vi "transconductance.vi"(6 "reverse flattening array?":bool, 10 "load data from file?":bool=TRUE, 11 "New Files to Process":string="\\G:\\My Drive\\ansom\\Data\\MNK\\SA03018F.20171127\\8 - sweep B, Vsg lockin\n\\G:\\My Drive\\ansom\\Data\\MNK\\SA03018F.20171127\\8A - sweep B, Vsg lockin\n\\G:\\My Drive\\ansom\\Data\\MNK\\SA03018F.20171127\\11 - sweep B, Vsg lockin\n\\G:\\My Drive\\ansom\\Data\\MNK\\SA03018F.20171127\\14 - sweep B, Vsg lockin, control\n\\G:\\My Drive\\ansom\\Data\\MNK\\SA03018F.20171127\\16A - sweep B, Vsg lockin, control\n\\G:\\My Drive\\ansom\\Data\\MNK\\SA03018F.20171127\\17A - sweep B, Vsg lockin, superlattice\nG:\\My Drive\\ansom\\Data\\MNK\\SA03018F.20171127\\17B - sweep B, Vsg lockin, superlattice\n\\G:\\My Drive\\ansom\\Data\\MNK\\SA03018F.20171127\\20A- sweep B, Vsg lockin, superlattice\n\\G:\\My Drive\\ansom\\Data\\MNK\\SA03018F.20171127\\20B- sweep B, Vsg lockin, superlattice\n\\G:\\My Drive\\ansom\\Data\\MNK\\SA03018F.20171127\\21 - sweep B, Vsg lockin, superlattice\n\\G:\\My Drive\\ansom\\Data\\MNK\\SA03018F.20171127\\27 - sweep B, Vsg lockin, superlattice\n\\G:\\My Drive\\ansom\\Data\\MNK\\SA03018F.20171127\\28 - sweep B, Vsg lockin, superlattice\n\\G:\\My Drive\\ansom\\Data\\MNK\\SA03018F.20171127\\30 A- sweep B, Vsg lockin, superlattice #1, 10 deg") -> (0 "N Array":T3(array[cluster])=[{"N1"=-18.0066, "N2"=0.0, "N3"=0.00010031838163786089, "N4"=-8.934251517959054e-06}, {"N1"=-18.0066, "N2"=0.0, "N3"=0.00010015710688317914, "N4"=-8.760468576758047e-06}, {"N1"=-17.8982, "N2"=0.0, "N3"=0.00010015658578170592, "N4"=-8.792187056308865e-06}, {"N1"=-17.7321, "N2"=0.0, "N3"=0.00010023617314889044, "N4"=-8.779868263484922e-06}, {"N1"=-17.5726, "N2"=0.0, "N3"=0.00010019995511560665, "N4"=-8.84165774395135e-06}, {"N1"=-17.4134, "N2"=0.0, "N3"=0.00010003346980786668, "N4"=-8.782458591171434e-06}, {"N1"=-17.2466, "N2"=0.0, "N3"=0.0001001851515834062, "N4"=-8.812405740457855e-06}, {"N1"=-17.0876, "N2"=0.0, "N3"=9.996424752835683e-05, "N4"=-8.954710552212481e-06}, {"N1"=-16.9281, "N2"=0.0, "N3"=0.00010007646623264942, "N4"=-8.854481733875301e-06}, {"N1"=-16.7606, "N2"=0.0, "N3"=0.00010004679822862351, "N4"=-8.981470131499153e-06}, {"N1"=-16.6009, "N2"=0.0, "N3"=0.0001003028451545284, "N4"=-8.871085764926499e-06}, {"N1"=-16.434, "N2"=0.0, "N3"=0.00010021984130505798, "N4"=-8.798917996142857e-06}, {"N1"=-16.2751, "N2"=0.0, "N3"=0.00010013678411204595, "N4"=-8.871536018707524e-06}, {"N1"=-16.1153, "N2"=0.0, "N3"=0.00010003739579812323, "N4"=-9.002633460435717e-06}, {"N1"=-15.9479, "N2"=0.0, "N3"=0.00010008052035782709, "N4"=-8.862463891358436e-06}, {"N1"=-15.7856, "N2"=0.0, "N3"=0.00010006900345905896, "N4"=-9.027597453519316e-06}, {"N1"=-15.6255, "N2"=0.0, "N3"=0.00010024796268127841, "N4"=-8.810080148087122e-06}, {"N1"=-15.4597, "N2"=0.0, "N3"=0.00010012278099735182, "N4"=-8.6648959751743e-06}, {"N1"=-15.2998, "N2"=0.0, "N3"=0.00010026276869148863, "N4"=-8.8579861832877e-06}, {"N1"=-15.1405, "N2"=0.0, "N3"=0.00010020886342342537, "N4"=-8.748208416016011e-06}, {"N1"=-14.9705, "N2"=0.0, "N3"=0.00010010848681985287, "N4"=-9.098051937499567e-06}, {"N1"=-14.8105, "N2"=0.0, "N3"=0.0001000699932307551, "N4"=-9.011246958484157e-06}, {"N1"=-14.6513, "N2"=0.0, "N3"=0.0001000757195132027, "N4"=-9.010900149672011e-06}, {"N1"=-14.4917, "N2"=0.0, "N3"=9.993824082988935e-05, "N4"=-9.002543121236742e-06}, {"N1"=-14.3289, "N2"=0.0, "N3"=0.00010010079768179213, "N4"=-8.847810640041594e-06}, {"N1"=-14.1729, "N2"=0.0, "N3"=0.00010001217031990934, "N4"=-8.969947764453797e-06}, {"N1"=-14.0128, "N2"=0.0, "N3"=0.00010007488582386121, "N4"=-8.784105469909449e-06}, {"N1"=-13.842, "N2"=0.0, "N3"=0.00010016251877130333, "N4"=-8.885939754527236e-06}, {"N1"=-13.6863, "N2"=0.0, "N3"=0.00010016244352366999, "N4"=-8.834835317879139e-06}, {"N1"=-13.5229, "N2"=0.0, "N3"=0.00010007728243774287, "N4"=-8.9305409259411e-06}, {"N1"=-13.3673, "N2"=0.0, "N3"=0.00010032215472754636, "N4"=-8.9276984567074e-06}, {"N1"=-13.201, "N2"=0.0, "N3"=0.0001000418821861951, "N4"=-8.845571431843766e-06}, {"N1"=-13.0442, "N2"=0.0, "N3"=0.00010004756843919491, "N4"=-8.832758065432273e-06}, {"N1"=-12.8839, "N2"=0.0, "N3"=0.00010011457464201885, "N4"=-8.909556350127235e-06}, {"N1"=-12.7138, "N2"=0.0, "N3"=9.990626272763215e-05, "N4"=-8.869462858430907e-06}, {"N1"=-12.55, "N2"=0.0, "N3"=0.0001001918886167206, "N4"=-8.814838476725855e-06}, {"N1"=-12.39, "N2"=0.0, "N3"=0.00010022579508319459, "N4"=-8.933618209144054e-06}, {"N1"=-12.2233, "N2"=0.0, "N3"=0.00010012664489283517, "N4"=-8.953911074665986e-06}, {"N1"=-12.063, "N2"=0.0, "N3"=0.00010017088260306728, "N4"=-8.575368278082284e-06}, {"N1"=-11.8971, "N2"=0.0, "N3"=0.00010004924130002626, "N4"=-8.77894302199666e-06}, {"N1"=-11.7303, "N2"=0.0, "N3"=0.00010002693396616548, "N4"=-8.567433901573686e-06}, {"N1"=-11.5705, "N2"=0.0, "N3"=0.00010010692966113871, "N4"=-8.644552988417748e-06}, {"N1"=-11.4075, "N2"=0.0, "N3"=0.00010024657294306636, "N4"=-8.88388168403566e-06}, {"N1"=-11.2413, "N2"=0.0, "N3"=0.00010009391644656561, "N4"=-8.811695071710696e-06}, {"N1"=-11.0812, "N2"=0.0, "N3"=0.00010019896444949645, "N4"=-8.845852023691481e-06}, {"N1"=-10.9145, "N2"=0.0, "N3"=0.00010005773249972667, "N4"=-8.844120130650792e-06}, {"N1"=-10.7549, "N2"=0.0, "N3"=0.00010018480166106833, "N4"=-8.679352901815746e-06}, {"N1"=-10.5953, "N2"=0.0, "N3"=0.0001000782830667455, "N4"=-8.76691599357836e-06}, {"N1"=-10.4249, "N2"=0.0, "N3"=9.993264798222509e-05, "N4"=-8.96504813464287e-06}, {"N1"=-10.2654, "N2"=0.0, "N3"=9.995433520835375e-05, "N4"=-8.968012967483327e-06}, {"N1"=-10.105, "N2"=0.0, "N3"=0.00010014526620665925, "N4"=-8.70639827930858e-06}, {"N1"=-9.9336, "N2"=0.0, "N3"=0.00010009516639935694, "N4"=-8.909066311145657e-06}, {"N1"=-9.7748, "N2"=0.0, "N3"=9.988598517222335e-05, "N4"=-8.881139507922535e-06}, {"N1"=-9.6111, "N2"=0.0, "N3"=0.00010033492937531955, "N4"=-8.561841464266133e-06}, {"N1"=-9.4488, "N2"=0.0, "N3"=0.0001000108439398465, "N4"=-9.000451691819498e-06}, {"N1"=-9.2888, "N2"=0.0, "N3"=0.00010029092857058395, "N4"=-8.775049213930287e-06}, {"N1"=-9.1222, "N2"=0.0, "N3"=0.00010000246282915645, "N4"=-8.695591943572876e-06}, {"N1"=-8.963, "N2"=0.0, "N3"=0.00010015749725789654, "N4"=-8.836612780808448e-06}, {"N1"=-8.8035, "N2"=0.0, "N3"=0.00010025081418287268, "N4"=-8.608048389168885e-06}, {"N1"=-8.6339, "N2"=0.0, "N3"=9.994809970083847e-05, "N4"=-8.730162238071121e-06}, {"N1"=-8.4707, "N2"=0.0, "N3"=0.00010002995161030842, "N4"=-9.020804557559828e-06}, {"N1"=-8.3074, "N2"=0.0, "N3"=0.0001002051806634715, "N4"=-8.804092790691239e-06}, {"N1"=-8.1512, "N2"=0.0, "N3"=0.00010013608964694704, "N4"=-8.657583789538865e-06}, {"N1"=-7.9883, "N2"=0.0, "N3"=0.00010004735386723776, "N4"=-8.797491651355247e-06}, {"N1"=-7.8245, "N2"=0.0, "N3"=0.00010011934839831245, "N4"=-8.693999817336747e-06}, {"N1"=-7.6575, "N2"=0.0, "N3"=0.00010009963923318637, "N4"=-8.920758810927737e-06}, {"N1"=-7.4903, "N2"=0.0, "N3"=0.00010008289455834287, "N4"=-8.891430231840132e-06}, {"N1"=-7.3313, "N2"=0.0, "N3"=0.00010026388542781577, "N4"=-8.870995927512986e-06}, {"N1"=-7.1681, "N2"=0.0, "N3"=0.00010005793665956295, "N4"=-8.785287793838638e-06}, {"N1"=-7.0116, "N2"=0.0, "N3"=0.00010012403992366044, "N4"=-9.084635578933354e-06}, {"N1"=-6.8517, "N2"=0.0, "N3"=0.00010018267176600397, "N4"=-8.7284533360535e-06}, {"N1"=-6.6921, "N2"=0.0, "N3"=0.00010011479820151499, "N4"=-8.752440206681594e-06}, {"N1"=-6.5291, "N2"=0.0, "N3"=0.00010022354549059768, "N4"=-8.696230423718127e-06}, {"N1"=-6.369, "N2"=0.0, "N3"=0.00010001230601861005, "N4"=-8.826376350692743e-06}, {"N1"=-6.2091, "N2"=0.0, "N3"=0.00010009635543729479, "N4"=-8.769349316099743e-06}, {"N1"=-6.0387, "N2"=0.0, "N3"=0.00010021713542801924, "N4"=-8.780040147694486e-06}, {"N1"=-5.8793, "N2"=0.0, "N3"=9.999814998298704e-05, "N4"=-8.789703944994364e-06}, {"N1"=-5.719, "N2"=0.0, "N3"=0.00010021176189713136, "N4"=-8.644330249039203e-06}, {"N1"=-5.5465, "N2"=0.0, "N3"=0.00010016910593251693, "N4"=-8.601585040210062e-06}, {"N1"=-5.3809, "N2"=0.0, "N3"=0.00010015154961593695, "N4"=-8.885007698359212e-06}, {"N1"=-5.221, "N2"=0.0, "N3"=0.00010018628999205372, "N4"=-8.75778968697093e-06}, {"N1"=-5.0615, "N2"=0.0, "N3"=0.00010011540589565727, "N4"=-8.787367507169681e-06}, {"N1"=-4.8915, "N2"=0.0, "N3"=0.00010013584944994493, "N4"=-8.761960490469314e-06}, {"N1"=-4.7348, "N2"=0.0, "N3"=0.00010028126497114088, "N4"=-8.768436572507557e-06}, {"N1"=-4.5716, "N2"=0.0, "N3"=0.0001002920507683757, "N4"=-8.867055108840846e-06}, {"N1"=-4.4114, "N2"=0.0, "N3"=0.00010008569235620579, "N4"=-8.545254799522978e-06}, {"N1"=-4.2446, "N2"=0.0, "N3"=0.00010012804807007648, "N4"=-8.897243918678671e-06}, {"N1"=-4.0845, "N2"=0.0, "N3"=0.00010009767215190891, "N4"=-8.677128466307431e-06}, {"N1"=-3.9168, "N2"=0.0, "N3"=0.00010017888369554464, "N4"=-8.724465870121636e-06}, {"N1"=-3.7502, "N2"=0.0, "N3"=0.00010012004211457495, "N4"=-8.880147453346872e-06}, {"N1"=-3.5873, "N2"=0.0, "N3"=0.0001000455164194285, "N4"=-8.568397424073202e-06}, {"N1"=-3.4201, "N2"=0.0, "N3"=0.00010005267050495742, "N4"=-8.973105346027973e-06}, {"N1"=-3.2605, "N2"=0.0, "N3"=0.00010011192632412391, "N4"=-8.78477028889865e-06}, {"N1"=-3.093, "N2"=0.0, "N3"=9.990616837060194e-05, "N4"=-8.775455280917142e-06}, {"N1"=-2.9338, "N2"=0.0, "N3"=0.00010005357240971674, "N4"=-8.615380984712672e-06}, {"N1"=-2.7728, "N2"=0.0, "N3"=0.00010019062986050772, "N4"=-8.804791976454716e-06}, {"N1"=-2.612, "N2"=0.0, "N3"=0.00010032559602195966, "N4"=-8.717347277962167e-06}, {"N1"=-2.4531, "N2"=0.0, "N3"=0.0001001875318509703, "N4"=-8.954695371795572e-06}, {"N1"=-2.283, "N2"=0.0, "N3"=0.0001003015301175533, "N4"=-8.73974357489087e-06}, {"N1"=-2.1239, "N2"=0.0, "N3"=0.00010009905479790773, "N4"=-8.807237913703172e-06}, {"N1"=-1.961, "N2"=0.0, "N3"=0.00010005818395495428, "N4"=-8.599503424039064e-06}, {"N1"=-1.8027, "N2"=0.0, "N3"=0.00010020103036406647, "N4"=-8.729450538156992e-06}, {"N1"=-1.6401, "N2"=0.0, "N3"=0.00010023639043504032, "N4"=-8.664602084985559e-06}, {"N1"=-1.4805, "N2"=0.0, "N3"=0.00010015782060339108, "N4"=-8.638333249873085e-06}, {"N1"=-1.3103, "N2"=0.0, "N3"=0.0001001269717458062, "N4"=-8.628006539838728e-06}, {"N1"=-1.1557, "N2"=0.0, "N3"=0.00010006040840392438, "N4"=-8.57525884480477e-06}, {"N1"=-0.993, "N2"=0.0, "N3"=0.00010003322669903495, "N4"=-8.575347329466473e-06}, {"N1"=-0.8347, "N2"=0.0, "N3"=0.00010008580604159302, "N4"=-8.549653343395372e-06}, {"N1"=-0.671, "N2"=0.0, "N3"=0.00010025609285596, "N4"=-8.690837539466247e-06}, {"N1"=-0.5093, "N2"=0.0, "N3"=0.00010016699228213113, "N4"=-8.960201722509074e-06}, {"N1"=-0.3496, "N2"=0.0, "N3"=0.00010001742035309772, "N4"=-8.594650685903775e-06}, {"N1"=-0.1882, "N2"=0.0, "N3"=0.00010006869372628791, "N4"=-8.663134329725862e-06}, {"N1"=-0.0293, "N2"=0.0, "N3"=0.00010013932692011866, "N4"=-8.667920508751497e-06}, {"N1"=0.0043, "N2"=0.0, "N3"=0.00010015805934131428, "N4"=-8.9335205480663e-06}], 1 "peak diff":T1(graph), 2 "adjusted trans":dbl[][](graph), 3 "Intensity Graph 12":dbl[][](graph), 8 "B max":dbl=0.0043, 9 "B min":dbl=-18.0066)   [LabVIEW 2016]
uses:
  <vilib>/Analysis/3filter.llb/Filter Passband Type.ctl
  <userlib>/_MGI/File/Spreadsheet/MGI Write Spreadsheet Behavior Enum.ctl
  <vilib>/Analysis/6fits.llb/Remove Outliers (Range).vi
  <vilib>/Analysis/2dsp.llb/Decimate (single shot, DBL).vi
  <vilib>/Analysis/3filter.llb/Chebyshev Filter (DBL).vi
  <vilib>/Analysis/NI_AAL_SigProc.lvlib
  Transconductance State Machine/Tranconductance SM.lvclass
  <vilib>/Analysis/NI_AALPro.lvlib
  <vilib>/Analysis/NI_AALBase.lvlib
panel:
  in  "low cutoff freq: fh 2":dbl=0.45000000000000007 format="%0.2f"
  in  "filter? 2":bool
  out "trans offset 3":T1(graph)
  in  "offset cond waterfall":dbl
  out "trans offset 2":T1(graph)
  out "Array 3":dbl[](array[numeric])=[-18.0066, -18.0066, -17.8982, -17.7321, -17.5726, -17.4134, -17.2466, -17.0876, -16.9281, -16.7606, -16.6009, -16.434, -16.2751, -16.1153, -15.9479, -15.7856, -15.6255, -15.4597, -15.2998, -15.1405, -14.9705, -14.8105, -14.6513, -14.4917, -14.3289, -14.1729, -14.0128, -13.842, -13.6863, -13.5229, -13.3673, -13.201, -13.0442, -12.8839, -12.7138, -12.55, -12.39, -12.2233, -12.063, -11.8971, -11.7303, -11.5705, -11.4075, -11.2413, -11.0812, -10.9145, -10.7549, -10.5953, -10.4249, -10.2654, -10.105, -9.9336, -9.7748, -9.6111, -9.4488, -9.2888, -9.1222, -8.963, -8.8035, -8.6339, -8.4707, -8.3074, -8.1512, -7.9883, -7.8245, -7.6575, -7.4903, -7.3313, -7.1681, -7.0116, -6.8517, -6.6921, -6.5291, -6.369, -6.2091, -6.0387, -5.8793, -5.719, -5.5465, -5.3809, -5.221, -5.0615, -4.8915, -4.7348, -4.5716, -4.4114, -4.2446, -4.0845, -3.9168, -3.7502, -3.5873, -3.4201, -3.2605, -3.093, -2.9338, -2.7728, -2.612, -2.4531, -2.283, -2.1239, -1.961, -1.8027, -1.6401, -1.4805, -1.3103, -1.1557, -0.993, -0.8347, -0.671, -0.5093, -0.3496, -0.1882, -0.0293, 0.0043]
  in  "Array 2":dbl[](array[numeric])
  out "Vsg step":dbl=0.0002500000000000002
  in  "index 2":T2={"x axis"=3, "N2"=19, "N3"=4, "N4"=5, "V1"=8, "V2"=4, "V3"=10, "V4"=13, "CURRENT"=6, "Vsg"=1}
  in  "Enum":enum16{"X channel", "R"}(ring)
  out "appended array":dbl[][](array[numeric])=[[-18.0, 0.0, 0.04446097771376061, 0.006021672221753718, 0.05048264993551433, 0.028668012751153764, 0.07312899046491438, 0.0791506626866681], [-18.0, 0.0, -0.056373846952509576, 0.0, -0.056373846952509576, 0.02837384695250958, -0.027999999999999997, -0.027999999999999997], [-18.0, 0.0, 0.049493162070211774, -0.10540543652633572, -0.05591227445612394, 0.02791227445612395, 0.07740543652633572, -0.027999999999999997], [-17.5, 0.0, 0.046129347373157784, -0.10121998396218526, -0.05509063658902748, 0.027090636589027484, 0.07321998396218526, -0.027999999999999997], [-17.5, 0.0, 0.043444342785976746, 0.005170422757169932, 0.04861476554314668, 0.02721189511240476, 0.0706562378983815, 0.07582666065555144], [-17.5, 0.0, 0.04287468999966031, 0.003956037939553569, 0.04683072793921388, 0.026384955831716968, 0.06925964583137728, 0.07321568377093085], [-17.0, 0.0, 0.04387717223391915, 0.017165681819542214, 0.06104285405346136, 0.026030357249898807, 0.06990752948381795, 0.08707321130336017], [-17.0, 0.0, 0.04293110930010949, 0.002522344705542842, 0.04545345400565233, 0.025369630134107136, 0.06830073943421662, 0.07082308413975946], [-17.0, 0.0, 0.04308300880388786, 0.015047188702242795, 0.05813019750613065, 0.0251462400425529, 0.06822924884644076, 0.08327643754868355], [-17.0, 0.0, 0.04252161354318537, -0.09514180417958899, -0.05262019063640362, 0.02462019063640362, 0.067141804179589, -0.027999999999999997], [-16.5, 0.0, 0.04216871341900782, -0.09425258136841834, -0.05208386794941052, 0.024083867949410524, 0.06625258136841834, -0.027999999999999997], [-16.5, 0.0, 0.04249659427363511, -0.09388723675868076, -0.05139064248504564, 0.023390642485045646, 0.06588723675868076, -0.027999999999999997], [-16.5, 0.0, 0.040983126212713605, 0.027963674362191923, 0.06894680057490553, 0.022933772324838075, 0.06391689853755168, 0.0918805728997436], [-16.0, 0.0, 0.040294065093512466, 0.031053733991536964, 0.07134779908504943, 0.022598881705561374, 0.06289294679907384, 0.0939466807906108], [-16.0, 0.0, 0.04049866632115953, -0.09050062212970124, -0.050001955808541707, 0.022001955808541706, 0.06250062212970124, -0.027999999999999997], [-16.0, 0.0, 0.04000531787292696, -0.08960675339936605, -0.04960143552643909, 0.021601435526439096, 0.061606753399366054, -0.027999999999999997], [-15.5, 0.0, 0.039414110417272, 0.008151468001337217, 0.047565578418609214, 0.02125190952117613, 0.060666019938448126, 0.06881748793978534], [-15.5, 0.0, 0.039572360118108135, -0.08834654551755772, -0.048774185399449596, 0.020774185399449595, 0.06034654551755773, -0.027999999999999997], [-15.5, 0.0, 0.038893889697359116, 0.03145204420090134, 0.07034593389826045, 0.020424450133720098, 0.05931833983107921, 0.09077038403198055], [-15.0, 0.0, 0.03870474172165947, -0.08660554273962037, -0.0479008010179609, 0.019900801017960906, 0.058605542739620375, -0.027999999999999997], [-15.0, 0.0, 0.0385109481058909, -0.08602683483942901, -0.047515886733538105, 0.01951588673353811, 0.05802683483942901, -0.027999999999999997], [-15.0, 0.0, 0.03774130079155265, 0.030551452952921165, 0.06829275374447381, 0.019268560323351447, 0.057009861114904095, 0.08756131406782526], [-14.5, 0.0, 0.037690260052266944, -0.08437506207921786, -0.04668480202695092, 0.01868480202695092, 0.056375062079217865, -0.027999999999999997], [-14.5, 0.0, 0.037426407867293635, 0.028802451847391483, 0.06622885971468512, 0.018349210737912198, 0.05577561860520583, 0.08457807045259731], [-14.5, 0.0, 0.036907325586644404, 0.037059485474777845, 0.07396681106142225, 0.018119350932428824, 0.055026676519073225, 0.09208616199385107], [-14.0, 0.0, 0.036295775832950884, 0.028723731574441642, 0.06501950740739253, 0.017508182801357422, 0.053803958634308306, 0.08252769020874995], [-14.0, 0.0, 0.03637742241789385, -0.0815498175658215, -0.045172395147927646, 0.017172395147927646, 0.05354981756582149, -0.027999999999999997], [-14.0, 0.0, 0.03597236981258607, 0.0068401099555525716, 0.04281247976813864, 0.016788040715268352, 0.05276041052785442, 0.05960052048340699], [-13.5, 0.0, 0.03597823335114367, 0.009264323660455251, 0.04524255701159892, 0.016542677409166793, 0.052520910760310464, 0.061785234420765715], [-13.5, 0.0, 0.03566410493977318, 0.013273469156751233, 0.04893757409652441, 0.016102754191048774, 0.05176685913082195, 0.06504032828757318], [-13.5, 0.0, 0.03495340266237865, 0.040761103638829094, 0.07571450630120774, 0.015678312535950555, 0.05063171519832921, 0.0913928188371583], [-13.0, 0.0, 0.034773104025620664, 0.012710472899794996, 0.04748357692541566, 0.015119035295290864, 0.04989213932091153, 0.06260261222070652], [-13.0, 0.0, 0.03454294786961758, 0.03502968760301974, 0.06957263547263731, 0.014791848293227253, 0.04933479616284483, 0.08436448376586457], [-13.0, 0.0, 0.03431536386739489, 0.03446794580304063, 0.06878330967043551, 0.01455317511678769, 0.04886853898418258, 0.0833364847872232], [-12.5, 0.0, 0.03393420556647725, 0.04224524984791973, 0.07617945541439698, 0.014078805380758551, 0.0480130109472358, 0.09025826079515553], [-12.5, 0.0, 0.03351665751640095, 0.0436864265687828, 0.07720308408518375, 0.013620157500051681, 0.04713681501645263, 0.09082324158523543], [-12.5, 0.0, 0.03309970867264065, 0.00770581533578843, 0.04080552400842908, 0.013300093650137595, 0.046399802322778246, 0.054105617658566675], [-12.0, 0.0, 0.032909810210727905, 0.04035959987828144, 0.07326941008900933, 0.012939450624380532, 0.04584926083510844, 0.08620886071338987], [-12.0, 0.0, 0.03289416179249914, 0.008611328231694082, 0.04150549002419322, 0.012644182923613433, 0.04553834471611257, 0.054149672947806655], [-12.0, 0.0, 0.03263762503250849, 0.010273091437663875, 0.04291071647017237, 0.012195948237336619, 0.04483357326984511, 0.05510666470750899], [-11.5, 0.0, 0.0322700945202293, 0.037478693739777316, 0.06974878826000662, 0.011870715231136043, 0.04414080975136535, 0.08161950349114266], [-11.5, 0.0, 0.032362606652672155, 0.006146461454333681, 0.038509068107005835, 0.011398035608501498, 0.043760642261173655, 0.049907103715507335], [-11.5, 0.0, 0.03188216939495373, 0.03852648189935309, 0.07040865129430682, 0.011148873716445596, 0.043031043111399325, 0.08155752501075242], [-11.0, 0.0, 0.031617624734476886, 0.03705364473632219, 0.06867126947079907, 0.010840423684177342, 0.04245804841865423, 0.07951169315497641], [-11.0, 0.0, 0.031536723776243426, 0.009863175440164594, 0.04139989921640802, 0.01040903171495184, 0.041945755491195266, 0.05180893093135986], [-11.0, 0.0, 0.031229660288727763, 0.02679667274219269, 0.05802633303092045, 0.010086557851786283, 0.04131621814051405, 0.06811289088270674], [-11.0, 0.0, 0.03097858323433299, 0.007226609639897186, 0.03820519287423017, 0.00965133737350091, 0.0406299206078339, 0.04785653024773109], [-10.5, 0.0, 0.030790267952404, 0.01054006719869853, 0.04133033515110253, 0.009266260997557327, 0.040056528949961326, 0.050596596148659856], [-10.5, 0.0, 0.030491444081275687, 0.00811387579874373, 0.03860531988001942, 0.008913075783567814, 0.0394045198648435, 0.04751839566358723], [-10.5, 0.0, 0.03013635862620256, 0.034658236489774494, 0.06479459511597706, 0.008534631716298719, 0.03867099034250128, 0.07332922683227577], [-10.0, 0.0, 0.029870138097126887, 0.033161585200730634, 0.06303172329785753, 0.00826037639381876, 0.03813051449094565, 0.07129209969167628], [-10.0, 0.0, 0.02964018752255273, 0.03888847868674942, 0.06852866620930215, 0.007853191752792697, 0.03749337927534543, 0.07638185796209485], [-10.0, 0.0, 0.02958194968359225, 0.010576238915951157, 0.040158188599543405, 0.007680537126040206, 0.037262486809632456, 0.04783872572558361], [-9.5, 0.0, 0.02895054547168147, 0.03532780361508146, 0.06427834908676293, 0.007407562612708304, 0.03635810808438977, 0.07168591169947124], [-9.5, 0.0, 0.02908139244168985, 0.01645277290794269, 0.04553416534963254, 0.007064893179293604, 0.03614628562098345, 0.05259905852892614], [-9.5, 0.0, 0.02913599024272885, 0.030417165452800043, 0.059553155695528895, 0.006788473114287235, 0.03592446335701609, 0.06634162880981613], [-9.0, 0.0, 0.028804794879402247, 0.021857335495489925, 0.05066213037489217, 0.006374967326277696, 0.03517976220567994, 0.05703709770116987], [-9.0, 0.0, 0.028107595566255715, 0.021262040207239978, 0.04936963577349569, 0.006161090258068172, 0.03426868582432389, 0.055530726031563865], [-9.0, 0.0, 0.028002012517935077, 0.02004458859838206, 0.04804660111631714, 0.00593402645440961, 0.033936038972344686, 0.05398062757072675], [-8.5, 0.0, 0.027681926816933017, 0.01874863874213066, 0.04643056555906368, 0.005365795450533601, 0.03304772226746662, 0.05179636100959728], [-8.5, 0.0, 0.027722870144628244, 0.02161992077967207, 0.049342790924300314, 0.0052184374914273635, 0.03294130763605561, 0.05456122841572768], [-8.5, 0.0, 0.02789773831601293, 0.0204873212738447, 0.04838505958985763, 0.004956385283271967, 0.0328541235992849, 0.0533414448731296], [-8.0, 0.0, 0.027694549160098482, 0.016800227947095576, 0.04449477710719406, 0.004605963675474027, 0.03230051283557251, 0.04910074078266809], [-8.0, 0.0, 0.027287903704956453, 0.020242829151946827, 0.047530732856903284, 0.004537685493819293, 0.03182558919877575, 0.052068418350722574], [-8.0, 0.0, 0.027029934094200132, 0.01344481599595003, 0.04047475009015016, 0.004123976283842783, 0.031153910378042916, 0.044598726373992946], [-7.5, 0.0, 0.02685464727903425, 0.010761141340719524, 0.03761578861975377, 0.004060303874873182, 0.03091495115390743, 0.041676092494626955], [-7.5, 0.0, 0.026479530091908746, 0.019068339724119306, 0.045547869816028055, 0.003750286915240696, 0.030229817007149443, 0.04929815673126875], [-7.5, 0.0, 0.02644676836176484, 0.009048673793903603, 0.03549544215566844, 0.0037613453263880595, 0.030208113688152897, 0.0392567874820565], [-7.0, 0.0, 0.006981093422593114, 0.019308936446995946, 0.02629002986958906, 0.0035387118868820118, 0.010519805309475126, 0.029828741756471072], [-7.0, 0.0, 0.006574148855503611, 0.019798624611440527, 0.02637277346694414, 0.0032977724376183695, 0.00987192129312198, 0.029670545904562508], [-7.0, 0.0, 0.025802721322569874, 0.014714404199671825, 0.0405171255222417, 0.0027994178144077984, 0.028602139136977674, 0.0433165433366495], [-6.5, 0.0, 0.025679060797231045, 0.01380615683343947, 0.03948521763067051, 0.002822508513554864, 0.02850156931078591, 0.04230772614422538], [-6.5, 0.0, 0.025235838781037273, 0.013323014644376418, 0.038558853425413694, 0.002124367155650761, 0.027360205936688035, 0.04068322058106445], [-6.5, 0.0, 0.025491276680206197, 0.01251712506875496, 0.03800840174896116, 0.0023383570631220164, 0.027829633743328214, 0.040346758812083175], [-6.0, 0.0, 0.024818278021756998, 0.012075119237023146, 0.036893397258780145, 0.002077194791041466, 0.026895472812798464, 0.03897059204982161], [-6.0, 0.0, 0.024030811879570478, 0.01000230399747332, 0.034033115877043794, 0.0015803858760034166, 0.025611197755573894, 0.035613501753047214], [-6.0, 0.0, 0.008401895877167873, 0.015565510376663056, 0.02396740625383093, 0.0018493402622483139, 0.010251236139416187, 0.025816746516079243], [-5.5, 0.0, 0.023441907958200697, 0.006266922947008837, 0.029708830905209534, 0.0015229012211126875, 0.024964809179313385, 0.03123173212632222], [-5.5, 0.0, 0.023119646753681354, 0.007744322065931602, 0.030863968819612956, 0.0014318095448709487, 0.024551456298552304, 0.032295778364483906], [-5.5, 0.0, 0.022963986181598277, 0.012606615164283363, 0.03557060134588164, 0.0013055713702423378, 0.024269557551840616, 0.03687617271612398], [-5.0, 0.0, 0.022600665308077448, 0.01228298745341191, 0.03488365276148936, 0.0009080305717901399, 0.023508695879867588, 0.0357916833332795], [-5.0, 0.0, 0.022634212770038433, 0.028682858260289417, 0.05131707103032785, 0.0007072361712512289, 0.02334144894128966, 0.05202430720157908], [-5.0, 0.0, 0.02172580081012611, 0.010235994782749787, 0.031961795592875895, 0.00032442605284910216, 0.02205022686297521, 0.032286221645725], [-4.5, 0.0, 0.0212112632544696, 0.010908903061286408, 0.03212016631575601, 0.0005519233732244016, 0.021763186627694, 0.03267208968898041], [-4.5, 0.0, 0.020426068964988508, 0.009335704977419333, 0.02976177394240784, -0.00017156405243531613, 0.020254504912553192, 0.029590209889972525], [-4.5, 0.0, 0.01983326087196112, 0.009755427465993796, 0.029588688337954916, 0.0002557027427263281, 0.020088963614687448, 0.029844391080681244], [-4.0, 0.0, 0.019792867071431738, 0.010172940345957199, 0.029965807417388936, -0.00020226098261003593, 0.019590606088821703, 0.029763546434778902], [-4.0, 0.0, 0.01922892215945343, 0.00814384344557928, 0.027372765605032708, -0.0006856564218716208, 0.018543265737581808, 0.026687109183161088], [-4.0, 0.0, 0.01926659628525604, 0.01472169528494725, 0.03398829157020329, -0.00018264398303592108, 0.01908395230222012, 0.03380564758716737], [-4.0, 0.0, 0.01740280635812061, 0.005350312827337441, 0.02275311918545805, -0.0006182134391910281, 0.016784592918929583, 0.022134905746267024], [-3.5, 0.0, 0.016615062465511955, 0.005208696126189825, 0.02182375859170178, -0.0010267632482994823, 0.015588299217212474, 0.0207969953434023], [-3.5, 0.0, 0.016115265062774938, 0.005166525687780119, 0.021281790750555057, -0.0010572941750333496, 0.015057970887741589, 0.020224496575521708], [-3.5, 0.0, 0.019652886628280693, 0.007227870611031088, 0.02688075723931178, -0.0013104660893090115, 0.01834242053897168, 0.02557029115000277], [-3.0, 0.0, 0.014532328027844914, 0.006640751609659344, 0.02117307963750426, -0.001333017422093915, 0.013199310605751, 0.019840062215410344], [-3.0, 0.0, 0.01644502761422095, 0.004611766817680215, 0.021056794431901164, -0.0013582268062168924, 0.015086800808004057, 0.019698567625684272], [-3.0, 0.0, 0.016329832467207626, 0.0038369074921044757, 0.0201667399593121, -0.0015701975822271323, 0.014759634884980492, 0.018596542377084968], [-2.5, 0.0, 0.013383421807595726, 0.005858185343775869, 0.019241607151371593, -0.001631182114653887, 0.011752239692941839, 0.017610425036717708], [-2.5, 0.0, 0.018076556829058683, 0.005771789687313785, 0.02384834651637247, -0.0012252938355925963, 0.016851262993466086, 0.02262305268077987], [-2.5, 0.0, 0.01739746081558673, 0.0005990796437144348, 0.017996540459301165, 0.004690344503685286, 0.022087805319272017, 0.022686884962986452], [-2.0, 0.0, 0.015952154409143795, 0.007479569887735443, 0.023431724296879237, 0.0042092520226684055, 0.0201614064318122, 0.027640976319547643], [-2.0, 0.0, 0.01078971031467579, 0.008785200989617102, 0.01957491130429289, 0.004017319484264722, 0.014807029798940512, 0.023592230788557614], [-2.0, 0.0, 0.012037913877487646, 0.0033201135921719534, 0.0153580274696596, 0.003297690299407882, 0.015335604176895529, 0.018655717769067482], [-1.5, 0.0, 0.009265054312053947, 0.009403516189821097, 0.018668570501875044, 0.0029143184999139956, 0.012179372811967942, 0.02158288900178904], [-1.5, 0.0, 0.011071943177444078, 0.0066323754264351956, 0.017704318603879273, 0.006825131185254007, 0.017897074362698086, 0.02452944978913328], [-1.5, 0.0, 0.00726571658079586, 0.006688919396363445, 0.013954635977159305, 0.005206229514683909, 0.01247194609547977, 0.019160865491843215], [-1.0, 0.0, 0.01565415947513673, 0.012743817434941514, 0.028397976910078244, 0.005411521455721667, 0.021065680930858397, 0.03380949836579991], [-1.0, 0.0, 0.006614821989102807, 0.00903761457393817, 0.015652436563040977, 0.005404201298515806, 0.012019023287618613, 0.021056637861556784], [-1.0, 0.0, 0.011063812315580623, 0.0026733256169105615, 0.013737137932491185, 0.011695714916480252, 0.022759527232060876, 0.025432852848971437], [-0.5, 0.0, 0.00950514563787488, 0.004467798773967746, 0.013972944411842625, 0.011036468035256436, 0.020541613673131315, 0.02500941244709906], [-0.5, 0.0, 0.011408870668572556, 0.006321790403900452, 0.01773066107247301, 0.01061625585440976, 0.022025126522982316, 0.028346916926882768], [-0.5, 0.0, 0.005426765416525366, 0.004900136065960629, 0.010326901482485995, 0.014643409430501634, 0.020070174847027, 0.02497031091298763], [-0.0, 0.0, 0.010120210471630203, 0.010723553923630835, 0.02084376439526104, 0.00877173688584145, 0.018891947357471652, 0.029615501281102487], [-0.0, 0.0, 0.008394141889680748, 0.005704751228936912, 0.01409889311861766, 0.008415338221328198, 0.016809480111008947, 0.02251423133994586], [0.0, 0.0, 0.0069729262894555645, 0.009339595423381718, 0.016312521712837282, 0.009815451048656856, 0.01678837733811242, 0.026127972761494138]] format="%#_4f"
  in  "Existing SS file":string
  in  "display graphs?":bool=TRUE
  in  "Path to spreadsheet file":path=path "P:/expt/Leiden MNK/SA02836H.20170110/processed/9-11-14-17-19A-25-38-40-41-42-43-44-45-46-47-48 _rounded _20-50-40.txt"
  in  "write SS file?":bool
  in  "Tab Control":T4(tab)=enum."offset trans"
  in  "X axis":enum16{"B field", "theta", "phi"}(ring)
  out "Conductance":T1(graph)
  out "Intensity Graph 14":dbl[][](graph)
  out "angle theta":dbl[](array[numeric])=[90.0, 90.0, 90.0, 90.0, 90.0, 90.0, 90.0, 90.0, 90.0, 90.0, 90.0, 90.0, 90.0, 90.0, 90.0, 90.0, 90.0, 90.0, 90.0, 90.0, 90.0, 90.0, 90.0, 90.0, 90.0, 90.0, 90.0, 90.0, 90.0, 90.0, 90.0, 90.0, 90.0, 90.0, 90.0, 90.0, 90.0, 90.0, 90.0, 90.0, 90.0, 90.0, 90.0, 90.0, 90.0, 90.0, 90.0, 90.0, 90.0, 90.0, 90.0, 90.0, 90.0, 90.0, 90.0, 90.0, 90.0, 90.0, 90.0, 90.0, 90.0, 90.0, 90.0, 90.0, 90.0, 90.0, 90.0, 90.0, 90.0, 90.0, 90.0, 90.0, 90.0, 90.0, 90.0, 90.0, 90.0, 90.0, 90.0, 90.0, 90.0, 90.0, 90.0, 90.0, 90.0, 90.0, 90.0, 90.0, 90.0, 90.0, 90.0, 90.0, 90.0, 90.0, 90.0, 90.0, 90.0, 90.0, 90.0, 90.0, 90.0, 90.0, 90.0, 90.0, 90.0, 90.0, 90.0, 90.0, 90.0, 90.0, 90.0, 90.0, 90.0, 90.0]
  out "angle phi":dbl[](array[numeric])=[95.08927612513106, 94.99878347427111, 95.01681602690836, 95.00586515694681, 95.0427263892153, 95.01742942759887, 95.02686734576112, 95.11884346969536, 95.05620173957512, 95.12984499771949, 95.05426028587105, 95.01748439141417, 95.06285407432057, 95.1423485862178, 95.06053221709402, 95.15491141455168, 95.02241486721714, 94.94620768789837, 95.04884230043261, 94.98925792111928, 95.19288513976323, 95.14557454919512, 95.1450847428335, 95.14737186056, 95.05119031596786, 95.12506337378304, 95.01629923447294, 95.0697351433238, 95.04073271438969, 95.0993646532378, 95.08537258026323, 95.05287711710149, 95.04531022782125, 95.08556024395727, 95.07329541453824, 95.02791156735047, 95.09359358366443, 95.11013126081596, 94.89301265836426, 95.0146446373503, 94.8955082177529, 94.93543016221378, 95.06433930703732, 95.03102213056931, 95.04515582357456, 95.05125621415058, 94.95136729190656, 95.00636377054254, 95.12633321253064, 95.12691280271886, 94.96866994162558, 95.08626285111079, 95.08096535051908, 94.87738287396493, 95.14246662314575, 95.00041382639081, 94.96958469821104, 95.04198932535171, 94.90767159424387, 94.99194231615333, 95.15305358492549, 95.02115094756621, 94.94140075824754, 95.0252799740982, 94.96290758569866, 95.0926767432988, 95.07686609933987, 95.05616311200129, 95.01781647705106, 95.18446819219609, 94.9793428406699, 94.99632549769876, 94.9590393103361, 95.04345219309504, 95.0068467081343, 95.00690878208289, 95.02331211323961, 94.9301662256994, 94.90798532859078, 95.06975845836735, 94.99581434573432, 95.01613191039432, 95.0006864261797, 94.9971437976943, 95.05251665237051, 94.8800434272183, 95.07788929692397, 94.9543919660618, 94.97726678261054, 95.06858592404912, 94.89515113287007, 95.12479363383466, 95.01483029423464, 95.0198043942764, 94.92146713858176, 95.02227322415841, 94.96598977266439, 95.10748708291422, 94.97987272866872, 95.02823357208027, 94.9122163341498, 94.97900103623942, 94.94046260224368, 94.92940306786065, 94.92504865830874, 94.89832643484634, 94.89970127406148, 94.88253769834466, 94.95437841967342, 95.1116535081757, 94.91144903833808, 94.94786669607679, 94.94711213835079, 95.09696475666159]
  in  "Range":dbl[](array[numeric])
  in  "dy/dx vs x":bool=TRUE
  in  "trans diff":dbl=15.0
  out "Transconductance":T1(graph)
  out "peak locations":T1(graph)
  out "adjusted transconductance 2":dbl[][](graph)
  out "grandconductance":dbl[][](graph)
  out "Grandconductance":T1(graph)
  in  "grand diff":dbl=20.0
  out "Flattened Transconductance":dbl[][](graph)
  out "adjusted transconductance":T1(graph)
  out "flattened and interpolated transconductance":T1(graph)
  in  "threshold":dbl=25.0 format="%0.2f"
  in  "X Step":dbl=0.00025 format="%#_13g"
  in  "X High":dbl=0.1 format="%#_13g"
  in  "X Low":dbl=-0.1 format="%#_13g"
  in  "Array":dbl[](array[numeric])=array[10001 elements] format="%0.5f"
  out "size(s)":i32=114
  in  "width":i32=20 min=3
  out "Flattened Transconductance Avg":dbl[][](graph)
  in  "avg intensity plot":i32
  in  "manual shift only":bool
  out "Waveform Graph":dbl[](graph)
  in  "threshold 2":dbl=25.0 format="%0.2f"
  in  "width 2":i32=25 min=3
  out "first peak":cluster{dbl[], "Best Linear Fit":dbl[]}[](graph)
  in  "index":i32
  in  "length":i32
  in  "X Low 3":dbl=-0.06 format="%#_13g"
  in  "X High 3":dbl=0.6 format="%#_13g"
  in  "X Step 3":dbl=0.002 format="%#_13g"
  in  "low cutoff freq: fl":dbl=0.04 format="%#_13g"
  in  "filter type":T5
  in  "high cutoff freq: fh":dbl=0.45000000000000007 format="%0.2f"
  in  "filter?":bool
  out "Waveform Graph 2":dbl[][](graph)
  in  "offset grand":dbl
  in  "offset trans":dbl=50.0
  out "cond offset":T1(graph)
  out "trans offset":T1(graph)
  in  "offset cond":dbl=-0.002
  in  "decimating factor":i32=10
  in  "offset trans 2":dbl=0.02
  in  "offset 2":dbl
  out "Y line cut 6":T1(graph)
  in  "offset 3":dbl=0.05
  out "flattened and interpolated transconductance 2":T1(graph)
  # "control: V1=14, V2=10, current=8\nsuperlattice: V1=8, V2=4, current=6"
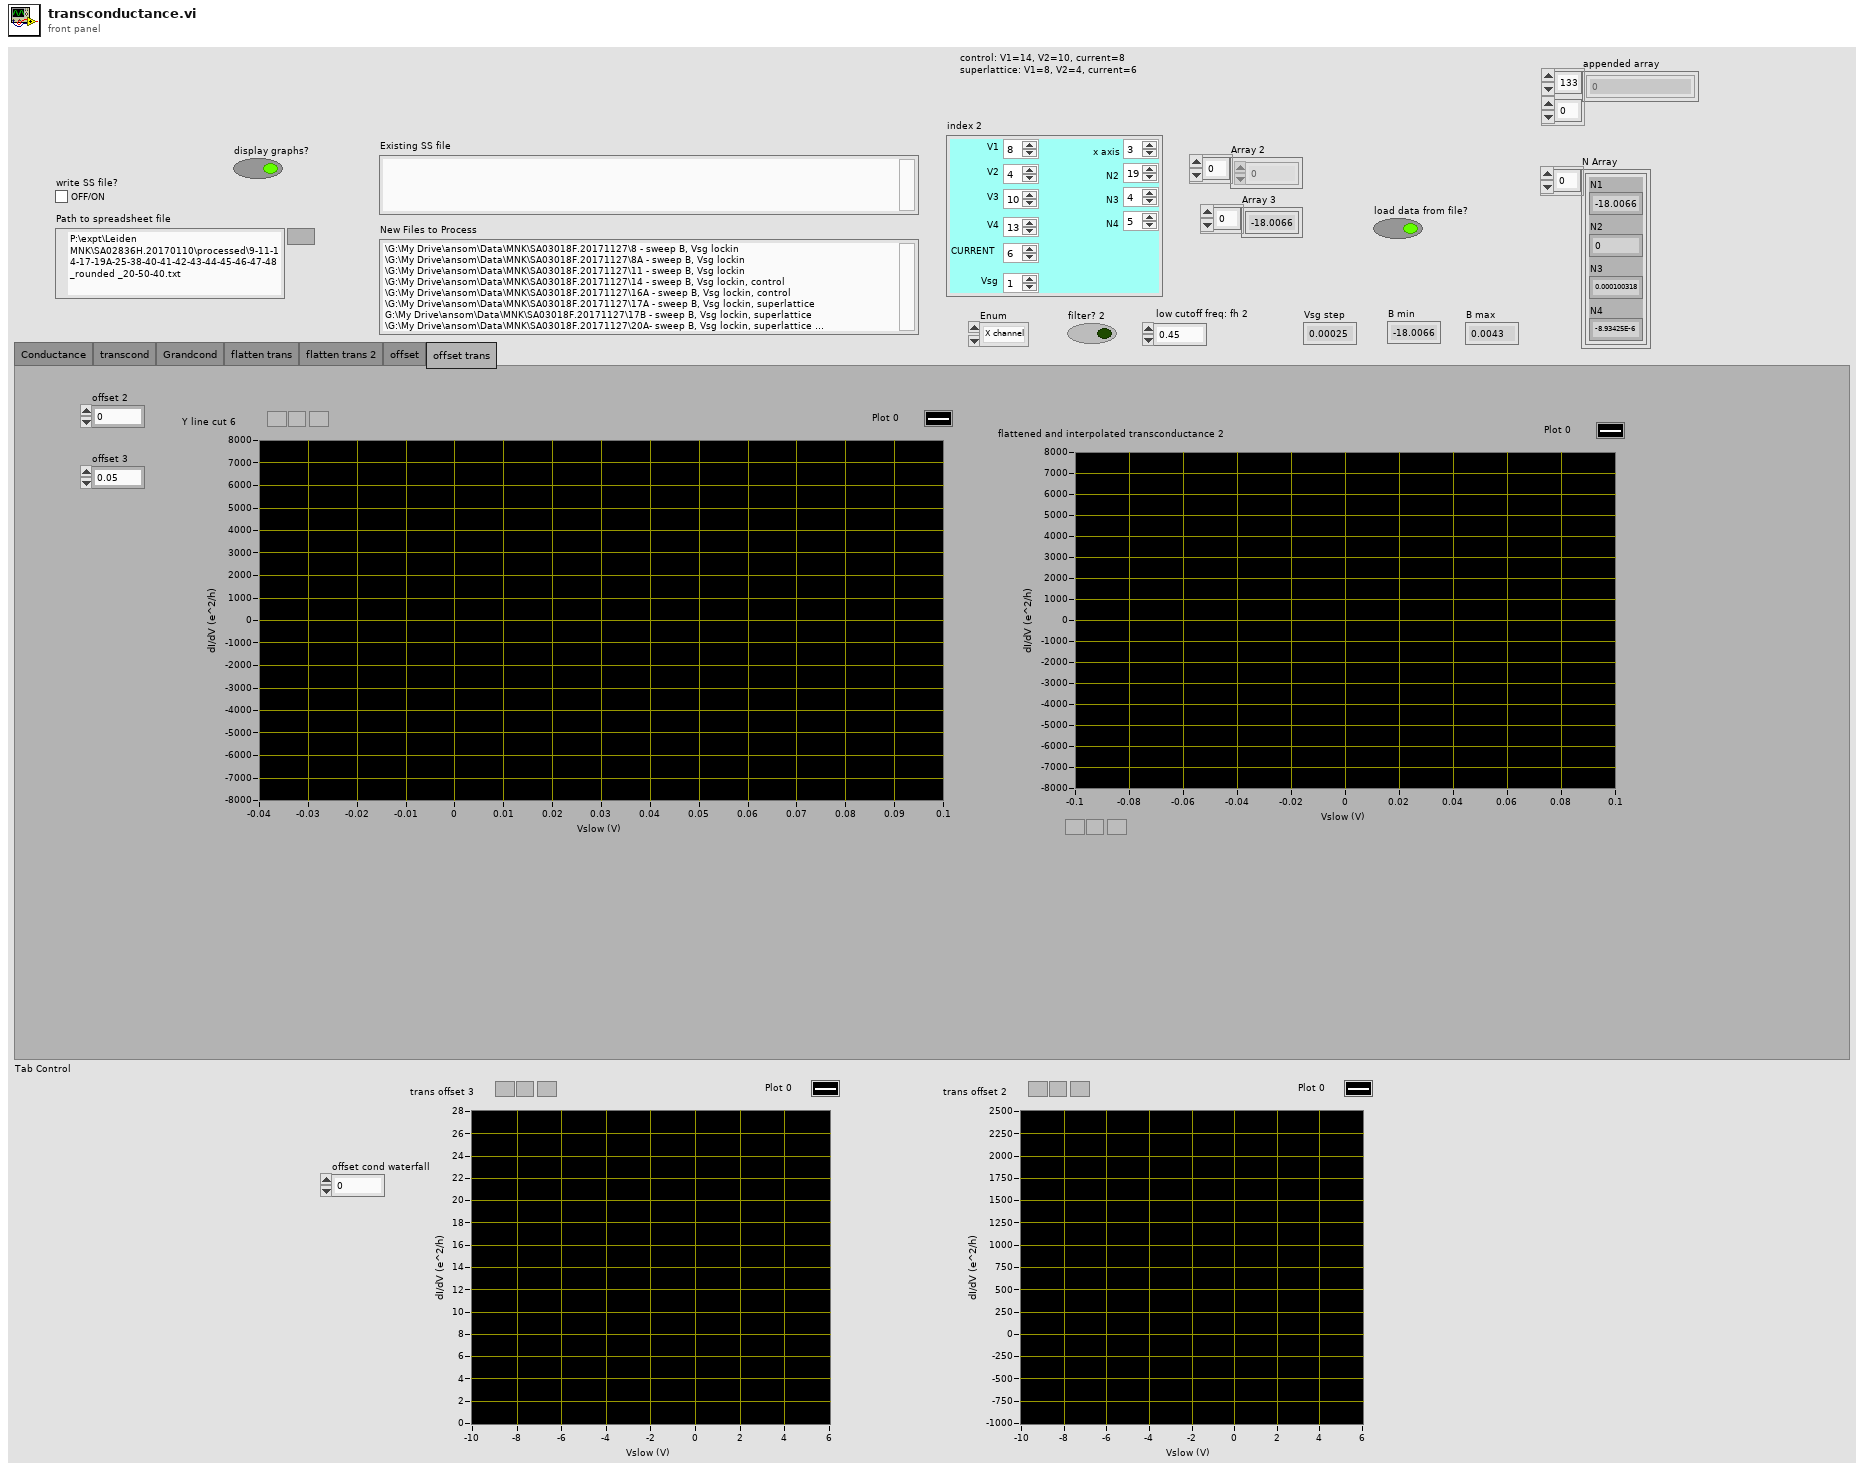
[diagram p1: front panel]
types:
  T1 = cluster{"Vfast":dbl[], "Decimated Array":dbl[]}[]
  T2 = cluster{"x axis":i32, "N2":i32, "N3":i32, "N4":i32, "V1":i32, "V2":i32, "V3":i32, "V4":i32, "CURRENT":i32, "Vsg":i32}
  T3 = cluster{"N1":dbl, "N2":dbl, "N3":dbl, "N4":dbl}[]
  T4 = enum32{"Conductance", "transcond", "Grandcond", "flatten trans", "flatten trans 2", "offset", "offset trans"}
  T5 = typedef "NI_AALBase.lvlib/Filter Passband Type.ctl" = enum32{"Lowpass", "Highpass", "Bandpass", "Bandstop"}
  T6 = cluster{"Decimated Array":dbl[], "Decimated Array":dbl[]}
  T7 = typedef "MGI Write Spreadsheet Behavior Enum.ctl" = enum16{"Append data", "Append headers and data", "Overwrite"}
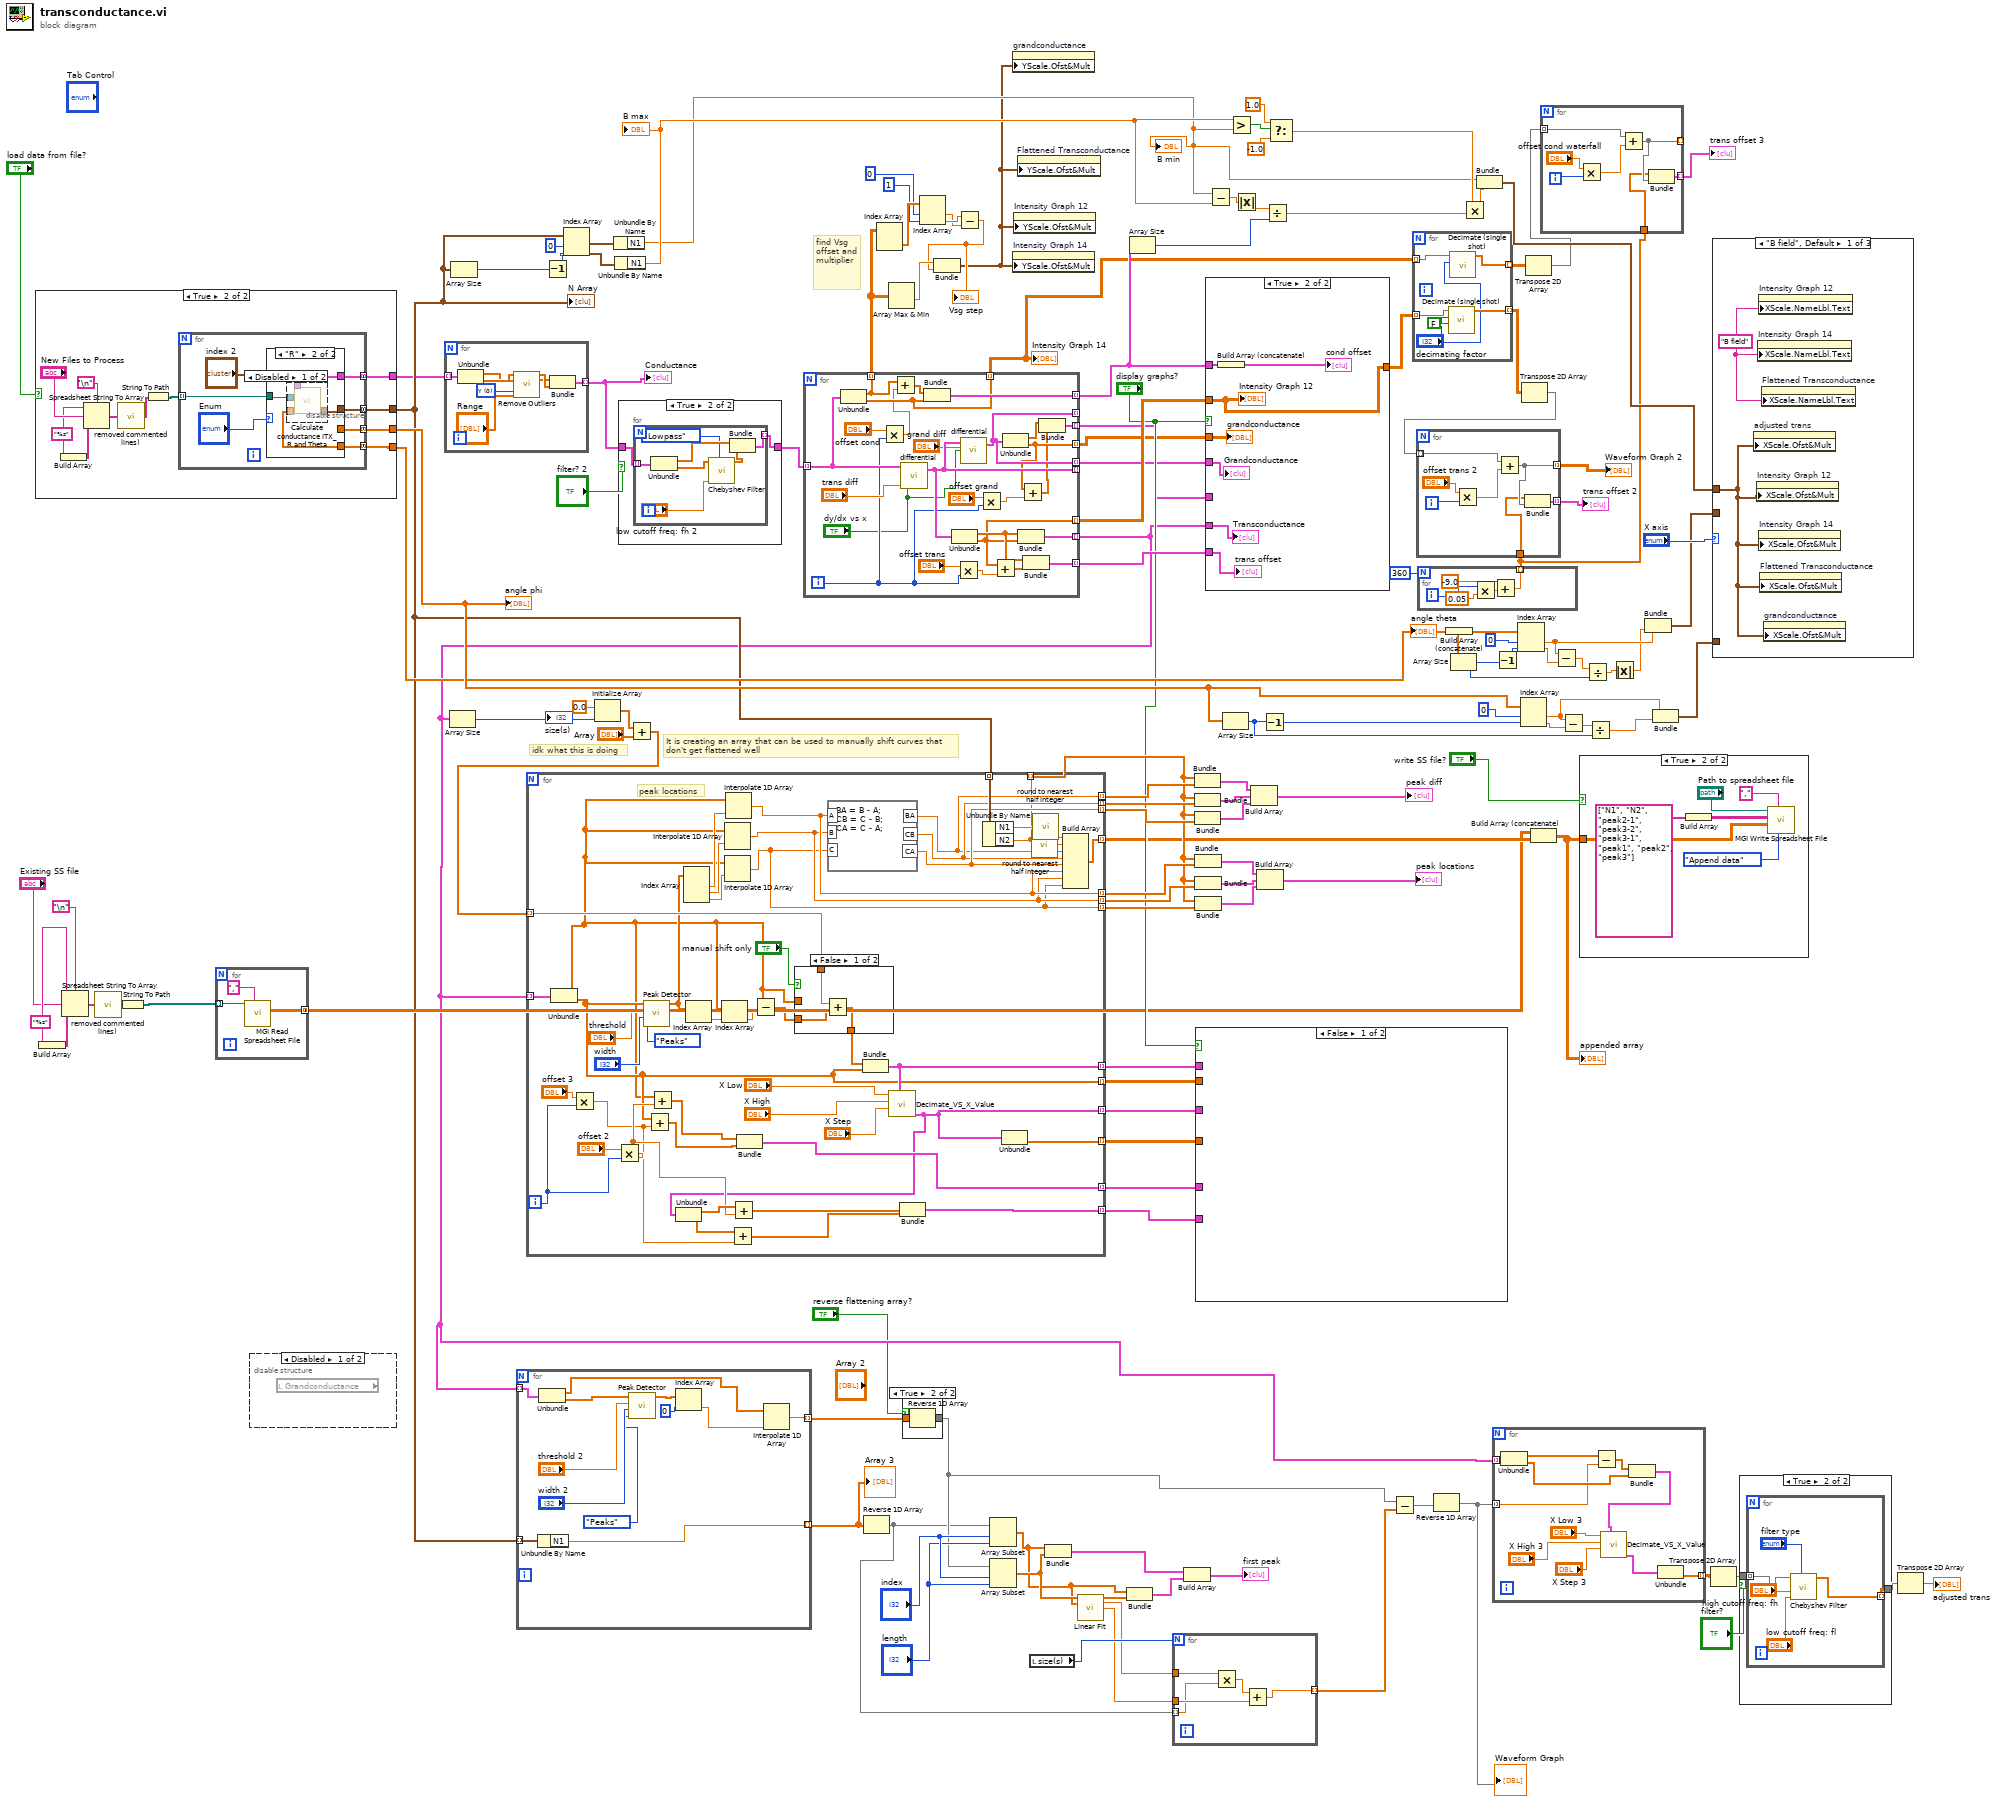
[diagram p0: block diagram]
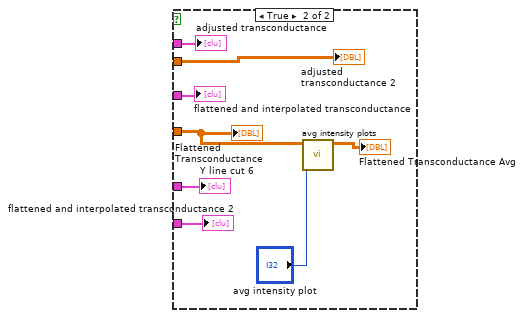
[diagram p6: hidden frame]
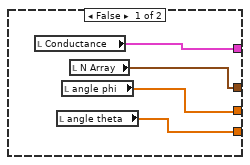
[diagram p9: hidden frame]
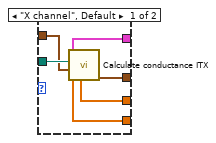
[diagram p10: hidden frame]
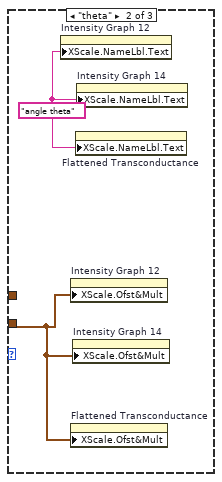
[diagram p12: hidden frame]
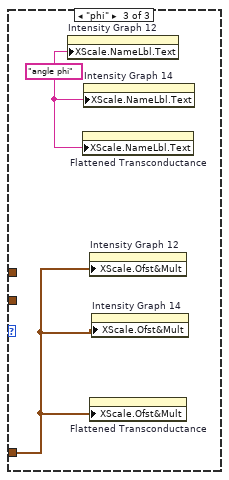
[diagram p13: hidden frame]
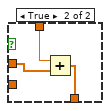
[diagram p14: hidden frame]
diagram:
  w48 = "%s" ("format string")
  # "It is creating an array that can be used to manually shift curves that\ndon't get flattened well"
  # "find Vsg offset and multiplier"
  # "idk what this is doing"
  n1 = case shown="True" "load data from file?" {
    tunnel: [w137 w148] -> w50
    tunnel: [w134 w147] -> w2
    tunnel: [w136 w146] -> w101
    tunnel: [w135 w145] -> w36
    frame False {
      n2 = local read "Conductance"() -> (w134:T1)
      n3 = local read "angle theta"() -> (w137:dbl[])
      n4 = local read "angle phi"() -> (w136:dbl[])
      n5 = local read "N Array"() -> (w135:T3)
    }
    frame True {
      w141 = "%s" ("format string")
      n6 = Build Array(w141) -> (w143:string[])
      n7 = Spreadsheet String To Array(delimiter (Tab)="\n", format string=w141, spreadsheet string="New Files to Process", array type (2D Dbl)=w143) -> (array=w139:string[])
      n8 = call "removed commented lines).vi"("Array in"=w139) -> ("Array out"=w138:string[])
      n9 = String To Path(string=w138) -> (path=w142:path[])
      n10 = for {
        tunnel: [w155] -> w147 mode=concatenating
        tunnel: [w154] -> w148 mode=concatenating
        tunnel: w142 -> [w153] mode=indexing
        tunnel: [w151] -> w146 mode=concatenating
        tunnel: [w152] -> w145 mode=concatenating
        n11 = case shown="\"R\"" "Enum" {
          tunnel: [w161 w164] -> w155
          tunnel: [w160 w162] -> w154
          tunnel: w153 -> [w159 w165]
          tunnel: [w158 w163] -> w152
          tunnel: [w157 _] -> w151
          tunnel: "index 2" -> [w156 _]
          frame "X channel", Default {
            n12 = call "Calculate conductance ITX.vi"("index"=w156, "File or Folder Path"=w159) -> ("N Array"=w158:T3, "angle phi"=w157:dbl[], "angle theta"=w160:dbl[], "A vs D"=w161:cluster{dbl[], dbl[]}[])  [unwired: 4 in, 2 out]
          }
          frame "R" {
            n13 = disable-structure shown="Disabled" {
              disable-tunnel: w165 -> [w169 _]
              disable-tunnel: [w168 _] -> w164
              disable-tunnel: [w167 _] -> w163
              disable-tunnel: [w166 _] -> w162
              frame Disabled {
                n14 = call "Calculate conductance ITX_R and Theta.vi"("File or Folder Path"=w169) -> ("N Array"=w167:T3, "angle theta"=w166:dbl[], "Resistance/Conductance vs Vsg"=w168:cluster{dbl[], dbl[]}[])  [unwired: 8 in]
              }
              frame Enabled {
              }
            }
          }
        }
      }
    }
  }
  "angle theta" <- w50
  "angle phi" <- w101
  "N Array" <- w36
  n15 = Build Array(w48) -> (w47:string[])
  n16 = Spreadsheet String To Array(delimiter (Tab)="\n", format string=w48, spreadsheet string="Existing SS file", array type (2D Dbl)=w47) -> (array=w40:string[])
  n17 = call "removed commented lines).vi"("Array in"=w40) -> ("Array out"=w39:string[])
  n18 = String To Path(string=w39) -> (path=w46:path[])
  n19 = for {
    tunnel: w46 -> [w172] mode=indexing
    tunnel: [w170] -> w41 mode=concatenating
    n20 = call <userlib>:"MGI Read Spreadsheet File.vi"("Delimiter (Tab)"=",", "Path"=w172) -> ("Values"=w170:dbl[][])  [unwired: 5 in, 4 out]
  }
  n21 = disable-structure shown="Disabled" {
    frame Disabled {
      n22 = local read "Grandconductance"() -> ()  [unwired: 1 out]
    }
    frame Enabled {
    }
  }
  n23 = for {
    tunnel: w2 -> [w180] mode=indexing
    tunnel: [w173] -> w1 mode=indexing
    w177 = u16 0 items=["Y", "X", "X and Y"] ("range type")
    n24 = Unbundle(w180) -> ("Vfast"=w178:dbl[], "Decimated Array"=w179:dbl[])
    n25 = call-poly <vilib>:"Remove Outliers.vi"("Y"=w179, "X"=w178, "range type"=w177, "Range"="Range") -> ("Y Out"=w175:dbl[], "X Out"=w174:dbl[])  [unwired: 7 in, 3 out]
    n26 = Bundle("X Out"=w174, "Y Out"=w175) -> (w173:cluster{"X Out":dbl[], "Y Out":dbl[]})  [unwired: 1 in]
  }
  "Conductance" <- w1
  n27 = Array Size(array=w36) -> (size(s)=w31:i32)
  n28 = Decrement(x=w31) -> (x-1=w30:i32)
  n29 = Index Array(array=w36, index #1=0 ("index"), index #2=w30) -> (element #1=w37:cluster{"N1":dbl, "N2":dbl, "N3":dbl, "N4":dbl}, element #2=w34:cluster{"N1":dbl, "N2":dbl, "N3":dbl, "N4":dbl})
  n30 = Unbundle By Name(w37) -> ("N1"=w32:dbl)
  "B min" <- w32
  n31 = Unbundle By Name(w34) -> ("N1"=w33:dbl)
  "B max" <- w33
  n32 = case shown="True" "filter? 2" {
    tunnel: w1 -> [w181 w183]
    tunnel: [w181 w182] -> w3
    frame False {
    }
    frame True {
      n33 = for {
        tunnel: w183 -> [w190] mode=indexing
        tunnel: [w186] -> w182 mode=indexing
        n34 = Unbundle(w190) -> ("X Out"=w187:dbl[], "Y Out"=w189:dbl[])
        n35 = call-poly <vilib>:"Chebyshev Filter.vi"("filter type"=Filter_Passband_Type."Lowpass", "low cutoff freq: fl"="low cutoff freq: fh 2", "X"=w189) -> ("Filtered X"=w188:dbl[])  [unwired: 7 in, 1 out]
        n36 = Bundle("X Out"=w187, "Filtered X"=w188) -> (w186:cluster{"X Out":dbl[], "Filtered X":dbl[]})  [unwired: 1 in]
      }
    }
  }
  n37 = for {
    tunnel: w3 -> [w213] mode=indexing
    tunnel: [w201] -> _ mode=indexing
    tunnel: [w214] -> w18 mode=indexing
    tunnel: [w202] -> w129 mode=indexing
    tunnel: [w212] -> w125 mode=indexing
    tunnel: [w210] -> w10 mode=indexing
    tunnel: [w209] -> w29 mode=indexing
    tunnel: [w205] -> w117 mode=indexing
    tunnel: [w196] -> w22 mode=indexing
    tunnel: [w200] -> _ mode=indexing
    tunnel: [w200] -> w21 mode=indexing
    tunnel: [w193] -> w20 mode=indexing
    i -> [w198]
    n38 = Unbundle(w213) -> ("X Out"=w209:dbl[], "Filtered X"=w210:dbl[])
    n39 = Multiply(x="offset cond", y=w198) -> (x*y=w203:dbl)
    n40 = Add(x=w209, y=w203) -> (x+y=w211:dbl[])
    n41 = call <userlib>:"differential.vi"("Numeric"="trans diff", "dy/dx vs x"="dy/dx vs x", "A vs B 2"=w213) -> ("A vs B 3"=w201:T6)  [unwired: 1 in]
    n42 = Bundle(w211, "Filtered X"=w210) -> (w212:cluster{dbl[], "Filtered X":dbl[]})  [unwired: 1 in]
    n43 = Unbundle(w201) -> ("Decimated Array"=w206:dbl[], "Decimated Array"=w202:dbl[])
    n44 = Multiply(x="offset trans", y=w198) -> (x*y=w208:dbl)
    n45 = call <userlib>:"differential.vi"("Numeric"="grand diff", "dy/dx vs x"="dy/dx vs x", "A vs B 2"=w201) -> ("A vs B 3"=w200:T6)  [unwired: 1 in]
    n46 = Multiply(x="offset grand", y=w198) -> (x*y=w197:dbl)
    n47 = Add(x=w202, y=w208) -> (x+y=w207:dbl[])
    n48 = Unbundle(w200) -> ("Decimated Array"=w195:dbl[], "Decimated Array"=w196:dbl[])
    n49 = Bundle("Decimated Array"=w206, "Decimated Array"=w202) -> (w214:T6)  [unwired: 1 in]
    n50 = Add(x=w196, y=w197) -> (x+y=w194:dbl[])
    n51 = Bundle("Decimated Array"=w206, w207) -> (w205:cluster{"Decimated Array":dbl[], dbl[]})  [unwired: 1 in]
    n52 = Bundle("Decimated Array"=w195, w194) -> (w193:cluster{"Decimated Array":dbl[], dbl[]})  [unwired: 1 in]
  }
  "Intensity Graph 14" <- w10
  n53 = Array Size(array=w18) -> (size(s)=w64:i32)
  "size(s)" <- w64
  n54 = for {
    tunnel: w18 -> [w228] mode=indexing
    tunnel: [w219] -> w5 mode=indexing
    tunnel: w36 -> [w223] mode=indexing
    tunnel: [w222] -> w94 mode=indexing
    n55 = Unbundle By Name(w223) -> ("N1"=w222:dbl)
    n56 = Unbundle(w228) -> ("Decimated Array"=w221:dbl[], "Decimated Array"=w217:dbl[])
    n57 = call <vilib>:"Peak Detector.vi"("peaks/valleys"=enum32{"Peaks", "Valleys"}."Peaks", "width"="width 2", "threshold"="threshold 2", "X"=w217) -> ("Locations"=w227:dbl[])  [unwired: 3 in, 4 out]
    n58 = Index Array(array=w227, index=0) -> (element=w220:dbl)
    n59 = Interpolate 1D Array(1:w220, 2:w221) -> (0:w219:dbl)
  }
  "Array 3" <- w94
  n60 = Initialize Array(0.0 ("element"), w64) -> (w57:dbl[])
  n61 = Add(x=w57, y="Array") -> (x+y=w55:dbl[])
  n62 = for {
    tunnel: [w251] -> w133 mode=indexing
    tunnel: [w250] -> w132 mode=indexing
    tunnel: [w269] -> w131 mode=indexing
    tunnel: w18 -> [w272] mode=indexing
    tunnel: w55 -> [w249] mode=indexing
    tunnel: [w266] -> w130 mode=indexing
    tunnel: [w262] -> w110 mode=indexing
    tunnel: [w239] -> w62 mode=indexing
    tunnel: [w238] -> w71 mode=indexing
    tunnel: [w237] -> w63 mode=indexing
    tunnel: w36 -> [w248] mode=indexing
    tunnel: [w255] -> w42 mode=indexing
    tunnel: [w240] -> w65 mode=indexing
    tunnel: [w245] -> w61 mode=indexing
    tunnel: [w246] -> w60 mode=indexing
    tunnel: [w247] -> w59 mode=indexing
    tunnel: [w232] -> w54 mode=indexing
    i -> [w265]
    # "peak locations"
    n63 = Unbundle(w272) -> ("Decimated Array"=w229:dbl[], "Decimated Array"=w240:dbl[])
    n64 = Multiply(x="offset 3", y=w265) -> (x*y=w258:dbl)
    n65 = Multiply(x="offset 2", y=w265) -> (x*y=w260:dbl)
    n66 = call <vilib>:"Peak Detector.vi"("peaks/valleys"=enum32{"Peaks", "Valleys"}."Peaks", "width"="width", "threshold"="threshold", "X"=w240) -> ("Locations"=w244:dbl[])  [unwired: 3 in, 4 out]
    n67 = Add(x=w240, y=w258) -> (x+y=w263:dbl[])
    n68 = Add(x=w229, y=w260) -> (x+y=w267:dbl[])
    n69 = Index Array(array=w244) -> (element #1=w243:dbl, element #2=w242:dbl, element #3=w241:dbl)  [unwired: 3 in]
    n70 = Index Array(array=w244) -> (element=w254:dbl)  [unwired: 1 in]
    n71 = Index Array(array=w229, index=w254) -> (element=w270:dbl)
    n72 = Interpolate 1D Array(1:w242, 2:w229) -> (0:w238:dbl)
    n73 = Interpolate 1D Array(1:w241, 2:w229) -> (0:w237:dbl)
    n74 = Interpolate 1D Array(1:w243, 2:w229) -> (0:w239:dbl)
    n75 = Bundle(w267, w263) -> (w266:cluster{dbl[], dbl[]})  [unwired: 1 in]
    n76 = Subtract(x=w229, y=w270) -> (x-y=w253:dbl[])
    n77 = case shown="False" "manual shift only" {
      tunnel: w253 -> [w277 _]
      tunnel: [w276 w281] -> w252
      tunnel: w249 -> [w278 w280]
      tunnel: w229 -> [_ w279]
      frame False {
        n78 = Add(x=w278, y=w277) -> (x+y=w276:dbl[])
      }
      frame True {
        n79 = Add(x=w280, y=w279) -> (x+y=w281:dbl[])
      }
    }
    n80 = formula code="BA = B - A;\nCB = C - B;\nCA = C - A;"("A"=w239, "B"=w238, "C"=w237) -> ("BA"=w245:dbl, "CB"=w246:dbl, "CA"=w247:dbl)
    n81 = Bundle(w252, "Decimated Array"=w240) -> (w251:cluster{dbl[], "Decimated Array":dbl[]})  [unwired: 1 in]
    n82 = call <userlib>:"Decimate_VS_X_Value.vi"("XY Graph kind 1"=w251, "X Step"="X Step", "X High"="X High", "X Low"="X Low") -> ("Interpolated"=w250:cluster{dbl[], dbl[]})  [unwired: 6 in, 1 out]
    n83 = Unbundle(w250) -> (w261:dbl[], w259:dbl[])
    n84 = Add(x=w259, y=w258) -> (x+y=w256:dbl[])
    n85 = Add(x=w261, y=w260) -> (x+y=w257:dbl[])
    n86 = Bundle(w257, w256) -> (w262:cluster{dbl[], dbl[]})  [unwired: 1 in]
    n87 = Unbundle By Name(w248) -> ("N1"=w234:dbl, "N2"=w232:dbl)
    n88 = Unbundle(w250) -> (w269:dbl[])  [unwired: 1 out]
    n89 = call "round to nearest half integer.vi"("Numeric"=w232) -> ("rounded to nearest 0.5"=w233:dbl)
    n90 = call "round to nearest half integer.vi"("Numeric"=w234) -> ("rounded to nearest 0.5"=w231:dbl)
    n91 = Build Array(w231, w233, w245, w246, w247, w239, w238, w237) -> (w255:dbl[])
  }
  n92 = Reverse 1D Array(array=w94) -> (reversed array=w80:dbl[])
  n93 = Index Array(array=w29) -> (element=w28:dbl[])  [unwired: 2 in]
  n94 = Array Max & Min(array=w29) -> (min value=w128:dbl)  [unwired: 3 out]
  n95 = case shown="True" "reverse flattening array?" {
    tunnel: w5 -> [w282 w284]
    tunnel: [w282 w283] -> w85
    frame False {
    }
    frame True {
      n96 = Reverse 1D Array(array=w284) -> (reversed array=w283:dbl[])
    }
  }
  n97 = Index Array(array=w28, index #1=0 ("index"), index #2=1 ("index")) -> (element #1=w24:dbl, element #2=w25:dbl)
  n98 = Subtract(x=w25, y=w24) -> (x-y=w23:dbl)
  "Vsg step" <- w23
  n99 = Bundle(w128, w23) -> (w19:cluster{dbl, dbl})  [unwired: 1 in]
  n100 = Array Subset(array=w80, index="index", length="length") -> (w82:dbl[])
  n101 = Array Subset(array=w85, index="index", length="length") -> (w83:dbl[])
  n102 = property on="grandconductance" class="IntGraph (strict)"("YScale.Ofst&Mult"=w19) -> ()  [unwired: 2 in, 2 out]
  n103 = property on="Intensity Graph 14" class="IntGraph (strict)"("YScale.Ofst&Mult"=w19) -> ()  [unwired: 2 in, 2 out]
  n104 = property on="Intensity Graph 12" class="IntGraph (strict)"("YScale.Ofst&Mult"=w19) -> ()  [unwired: 2 in, 2 out]
  n105 = property on="Flattened Transconductance" class="IntGraph (strict)"("YScale.Ofst&Mult"=w19) -> ()  [unwired: 2 in, 2 out]
  n106 = local read "size(s)"() -> (w87:i32)
  n107 = Bundle(w82, w83) -> (w91:cluster{dbl[], dbl[]})  [unwired: 1 in]
  n108 = call <vilib>:"Linear Fit.vi"("Y"=w83, "X"=w82) -> ("Best Linear Fit"=w88:dbl[], "slope"=w84:dbl, "intercept"=w81:dbl)  [unwired: 9 in, 2 out]
  n109 = Bundle(w82, "Best Linear Fit"=w88) -> (w89:cluster{dbl[], "Best Linear Fit":dbl[]})  [unwired: 1 in]
  n110 = Array Size(array=w125) -> (size(s)=w124:i32)
  n111 = for {
    N: w87 -> [_]
    tunnel: w84 -> [w289]
    tunnel: w81 -> [w287]
    tunnel: [w286] -> w86 mode=indexing
    tunnel: w80 -> [w285] mode=indexing
    n112 = Multiply(x=w289, y=w285) -> (x*y=w288:dbl)
    n113 = Add(x=w288, y=w287) -> (x+y=w286:dbl)
  }
  n114 = Build Array(w91, w89) -> (→"first peak":cluster{dbl[], "Best Linear Fit":dbl[]}[])
  n115 = Bundle(w54, w61) -> (w73:cluster{dbl[], dbl[]})  [unwired: 1 in]
  n116 = Bundle(w54, w60) -> (w72:cluster{dbl[], dbl[]})  [unwired: 1 in]
  n117 = Bundle(w54, w59) -> (w66:cluster{dbl[], dbl[]})  [unwired: 1 in]
  n118 = Bundle(w54, w62) -> (w70:cluster{dbl[], dbl[]})  [unwired: 1 in]
  n119 = Bundle(w54, w71) -> (w69:cluster{dbl[], dbl[]})  [unwired: 1 in]
  n120 = Bundle(w54, w63) -> (w68:cluster{dbl[], dbl[]})  [unwired: 1 in]
  n121 = case shown="False" "display graphs?" {
    tunnel: w133 -> [_ w297]
    tunnel: w132 -> [_ w296]
    tunnel: w131 -> [_ w292]
    tunnel: w130 -> [_ w295]
    tunnel: w110 -> [_ w294]
    tunnel: w65 -> [_ w293]
    frame False {
    }
    frame True {
      n122 = call "avg intensity plots.vi"("length"="avg intensity plot", "Intensity Graph 12"=w292) -> ("Intensity Graph 13"=→"Flattened Transconductance Avg":dbl[][])  [unwired: 9 in]
      "Flattened Transconductance" <- w292
      "adjusted transconductance" <- w297
      "flattened and interpolated transconductance" <- w296
      "Y line cut 6" <- w295
      "flattened and interpolated transconductance 2" <- w294
      "adjusted transconductance 2" <- w293
    }
  }
  n123 = case shown="True" "display graphs?" {
    tunnel: w129 -> [_ w300]
    tunnel: w125 -> [_ w299]
    tunnel: w117 -> [_ w304]
    tunnel: w18 -> [_ w303]
    tunnel: w22 -> [_ w302]
    tunnel: w21 -> [_ w301]
    tunnel: w20 -> [_ _]
    tunnel: [_ w300] -> w16
    frame False {
    }
    frame True {
      n124 = Build Array (concatenate)(w299) -> (→"cond offset":cluster{dbl[], "Filtered X":dbl[]}[])
      "Transconductance" <- w303
      "Intensity Graph 12" <- w300
      "trans offset" <- w304
      "grandconductance" <- w302
      "Grandconductance" <- w301
    }
  }
  n125 = Subtract(x=w32, y=w33) -> (x-y=w127:dbl)
  n126 = Array Size(array=w101) -> (size(s)=w99:i32)
  n127 = Greater?(x=w33, y=w32) -> (0:w123:bool)
  n128 = Absolute Value(x=w127) -> (abs(x)=w126:dbl)
  n129 = Build Array(w73, w72, w66) -> (→"peak diff":cluster{dbl[], dbl[]}[])
  n130 = Build Array(w70, w69, w68) -> (→"peak locations":cluster{dbl[], dbl[]}[])
  n131 = Decrement(x=w99) -> (x-1=w100:i32)
  n132 = Divide(x=w126, y=w124) -> (x/y=w120:dbl)
  n133 = Select(t=1.0, s=w123, f=-1.0) -> (s? t:f=w119:dbl)
  n134 = Subtract(x=w85, y=w86) -> (x-y=w79:dbl[])
  n135 = for {
    tunnel: w16 -> [w310] mode=indexing
    tunnel: [w308] -> w14 mode=indexing
    tunnel: w10 -> [w307] mode=indexing
    tunnel: [w306] -> w9 mode=indexing
    n136 = call-poly <vilib>:"Decimate (single shot).vi"("averaging"=FALSE, "decimating factor"="decimating factor", "X"=w310) -> ("Decimated Array"=w308:dbl[])  [unwired: 7 in, 1 out]
    n137 = call-poly <vilib>:"Decimate (single shot).vi"("decimating factor"="decimating factor", "X"=w307) -> ("Decimated Array"=w306:dbl[])  [unwired: 8 in, 1 out]
  }
  n138 = for {
    N: 360 -> [_]
    tunnel: [w311] -> w7 mode=indexing
    i -> [w312]
    n139 = Multiply(x=w312, y=0.05) -> (x*y=w315:dbl)
    n140 = Add(x=-9.0, y=w315) -> (x+y=w311:dbl)
  }
  n141 = Reverse 1D Array(array=w79) -> (reversed array=w78:dbl[])
  "Waveform Graph" <- w78
  n142 = Build Array (concatenate)(w50) -> (w52:dbl[])
  n143 = Array Size(array=w52) -> (size(s)=w103:i32)
  n144 = Multiply(x=w119, y=w120) -> (x*y=w118:dbl)
  n145 = Bundle("N1"=w32, w118) -> (w115:cluster{"N1":dbl, dbl})  [unwired: 1 in]
  n146 = for {
    tunnel: w18 -> [w326] mode=indexing
    tunnel: [w319] -> w77 mode=indexing
    tunnel: w78 -> [w316] mode=indexing
    n147 = Unbundle(w326) -> ("Decimated Array"=w317:dbl[], "Decimated Array"=w325:dbl[])
    n148 = Subtract(x=w317, y=w316) -> (x-y=w318:dbl[])
    n149 = Bundle(w318, "Decimated Array"=w325) -> (w320:cluster{dbl[], "Decimated Array":dbl[]})  [unwired: 1 in]
    n150 = call <userlib>:"Decimate_VS_X_Value.vi"("XY Graph kind 1"=w320, "X Step"="X Step 3", "X High"="X High 3", "X Low"="X Low 3") -> ("Interpolated"=w321:cluster{dbl[], dbl[]})  [unwired: 6 in, 1 out]
    n151 = Unbundle(w321) -> (w319:dbl[])  [unwired: 1 out]
  }
  n152 = Decrement(x=w103) -> (x-1=w105:i32)
  n153 = Index Array(array=w52, index #1=0 ("index"), index #2=w105) -> (element #1=w114:dbl, element #2=w113:dbl)
  n154 = Index Array(array=w101, index #1=0 ("index"), index #2=w100) -> (element #1=w97:dbl, element #2=w96:dbl)
  n155 = Transpose 2D Array(2D array=w14) -> (transposed array=w11:dbl[][])
  n156 = for {
    tunnel: w11 -> [w331] mode=indexing
    tunnel: [w329] -> w15 mode=indexing
    tunnel: [w328] -> w13 mode=indexing
    tunnel: w7 -> [w327]
    i -> [w330]
    n157 = Multiply(x="offset trans 2", y=w330) -> (x*y=w332:dbl)
    n158 = Add(x=w331, y=w332) -> (x+y=w329:dbl[])
    n159 = Bundle(w327, w329) -> (w328:cluster{dbl[], dbl[]})  [unwired: 1 in]
  }
  "Waveform Graph 2" <- w15
  "trans offset 2" <- w13
  n160 = Transpose 2D Array(2D array=w9) -> (transposed array=w8:dbl[][])
  n161 = Build Array (concatenate)(w41, w42) -> (w44:dbl[][])
  "appended array" <- w44
  n162 = for {
    tunnel: w8 -> [w338] mode=indexing
    tunnel: [w336] -> _ mode=indexing
    tunnel: [w335] -> w6 mode=indexing
    tunnel: w7 -> [w334]
    i -> [w337]
    n163 = Multiply(x="offset cond waterfall", y=w337) -> (x*y=w339:dbl)
    n164 = Add(x=w338, y=w339) -> (x+y=w336:dbl[])
    n165 = Bundle(w334, w336) -> (w335:cluster{dbl[], dbl[]})  [unwired: 1 in]
  }
  "trans offset 3" <- w6
  n166 = Subtract(x=w114, y=w113) -> (x-y=w109:dbl)
  n167 = Subtract(x=w97, y=w96) -> (x-y=w104:dbl)
  n168 = case shown="True" "write SS file?" {
    tunnel: w44 -> [_ w344]
    frame False {
    }
    frame True {
      n169 = Build Array(string[] ["N1", "N2", "peak2-1", "peak3-2", "peak3-1", "peak1", "peak2", "peak3"] ("Header Lines[row][col]")) -> (w343:string[][])
      n170 = call <userlib>:"MGI Write Spreadsheet File.vi"("Existing File Behavior"=MGI_Write_Spreadsheet_Behavior_Enum."Append data", "Delimiter (Tab)"=",", "Data[row][col]"=w344, "Header Lines[row][col]"=w343, "Path"="Path to spreadsheet file") -> ()  [unwired: 3 in, 4 out]
    }
  }
  n171 = Divide(x=w109, y=w103) -> (x/y=w108:dbl)
  n172 = Divide(x=w104, y=w99) -> (x/y=w95:dbl)
  n173 = Absolute Value(x=w108) -> (abs(x)=w112:dbl)
  n174 = Bundle(w114, w112) -> (w111:cluster{dbl, dbl})  [unwired: 1 in]
  n175 = Bundle(w97, w95) -> (w102:cluster{dbl, dbl})  [unwired: 1 in]
  n176 = Transpose 2D Array(2D array=w77) -> (transposed array=w76:dbl[][])
  n177 = case shown="\"B field\", Default" "X axis" {
    tunnel: w115 -> [w347 _ _]
    tunnel: w111 -> [_ w350 _]
    tunnel: w102 -> [_ _ w352]
    frame "B field", Default {
      w348 = "B field"
      n178 = property on="adjusted trans" class="IntGraph (strict)"("XScale.Ofst&Mult"=w347) -> ()  [unwired: 2 in, 2 out]
      n179 = property on="Intensity Graph 12" class="IntGraph (strict)"("XScale.Ofst&Mult"=w347) -> ()  [unwired: 2 in, 2 out]
      n180 = property on="Intensity Graph 14" class="IntGraph (strict)"("XScale.NameLbl.Text"=w348) -> ()  [unwired: 2 in, 2 out]
      n181 = property on="Intensity Graph 12" class="IntGraph (strict)"("XScale.NameLbl.Text"=w348) -> ()  [unwired: 2 in, 2 out]
      n182 = property on="Intensity Graph 14" class="IntGraph (strict)"("XScale.Ofst&Mult"=w347) -> ()  [unwired: 2 in, 2 out]
      n183 = property on="Flattened Transconductance" class="IntGraph (strict)"("XScale.Ofst&Mult"=w347) -> ()  [unwired: 2 in, 2 out]
      n184 = property on="Flattened Transconductance" class="IntGraph (strict)"("XScale.NameLbl.Text"=w348) -> ()  [unwired: 2 in, 2 out]
      n185 = property on="grandconductance" class="IntGraph (strict)"("XScale.Ofst&Mult"=w347) -> ()  [unwired: 2 in, 2 out]
    }
    frame "theta" {
      w349 = "angle theta"
      n186 = property on="Intensity Graph 12" class="IntGraph (strict)"("XScale.NameLbl.Text"=w349) -> ()  [unwired: 2 in, 2 out]
      n187 = property on="Intensity Graph 12" class="IntGraph (strict)"("XScale.Ofst&Mult"=w350) -> ()  [unwired: 2 in, 2 out]
      n188 = property on="Flattened Transconductance" class="IntGraph (strict)"("XScale.Ofst&Mult"=w350) -> ()  [unwired: 2 in, 2 out]
      n189 = property on="Intensity Graph 14" class="IntGraph (strict)"("XScale.Ofst&Mult"=w350) -> ()  [unwired: 2 in, 2 out]
      n190 = property on="Flattened Transconductance" class="IntGraph (strict)"("XScale.NameLbl.Text"=w349) -> ()  [unwired: 2 in, 2 out]
      n191 = property on="Intensity Graph 14" class="IntGraph (strict)"("XScale.NameLbl.Text"=w349) -> ()  [unwired: 2 in, 2 out]
    }
    frame "phi" {
      w351 = "angle phi"
      n192 = property on="Intensity Graph 12" class="IntGraph (strict)"("XScale.NameLbl.Text"=w351) -> ()  [unwired: 2 in, 2 out]
      n193 = property on="Flattened Transconductance" class="IntGraph (strict)"("XScale.NameLbl.Text"=w351) -> ()  [unwired: 2 in, 2 out]
      n194 = property on="Intensity Graph 14" class="IntGraph (strict)"("XScale.NameLbl.Text"=w351) -> ()  [unwired: 2 in, 2 out]
      n195 = property on="Intensity Graph 12" class="IntGraph (strict)"("XScale.Ofst&Mult"=w352) -> ()  [unwired: 2 in, 2 out]
      n196 = property on="Flattened Transconductance" class="IntGraph (strict)"("XScale.Ofst&Mult"=w352) -> ()  [unwired: 2 in, 2 out]
      n197 = property on="Intensity Graph 14" class="IntGraph (strict)"("XScale.Ofst&Mult"=w352) -> ()  [unwired: 2 in, 2 out]
    }
  }
  n198 = case shown="True" "filter?" {
    tunnel: w76 -> [w353 w355]
    tunnel: [w353 w354] -> w75
    frame False {
    }
    frame True {
      n199 = for {
        tunnel: w355 -> [w359] mode=indexing
        tunnel: [w358] -> w354 mode=indexing
        n200 = call-poly <vilib>:"Chebyshev Filter.vi"("filter type"="filter type", "low cutoff freq: fl"="low cutoff freq: fl", "high cutoff freq: fh"="high cutoff freq: fh", "X"=w359) -> ("Filtered X"=w358:dbl[])  [unwired: 6 in, 1 out]
      }
    }
  }
  n201 = Transpose 2D Array(2D array=w75) -> (transposed array=→"adjusted trans":dbl[][])
